vi "lab1.vi"() -> ()   [LabVIEW 2018]
uses:
  <vilib>/Utility/file.llb/Read Delimited Spreadsheet (DBL).vi
  <vilib>/Utility/file.llb/Write Delimited Spreadsheet (DBL).vi
panel:
  in  "Path 2":path
  in  "Path":path
  out "XY Graph":cluster{"all rows":dbl[], "all rows":dbl[]}[](graph)
  out "Waveform Graph 3":cluster{i32, i32, "all rows":dbl[]}(graph)
  out "Waveform Graph":cluster{i32, i32, "all rows":dbl[]}(graph)
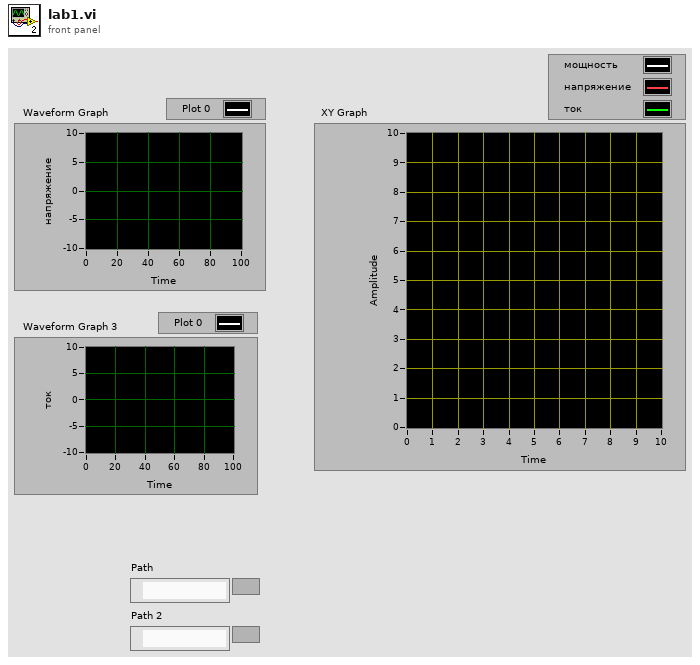
[diagram p1: front panel]
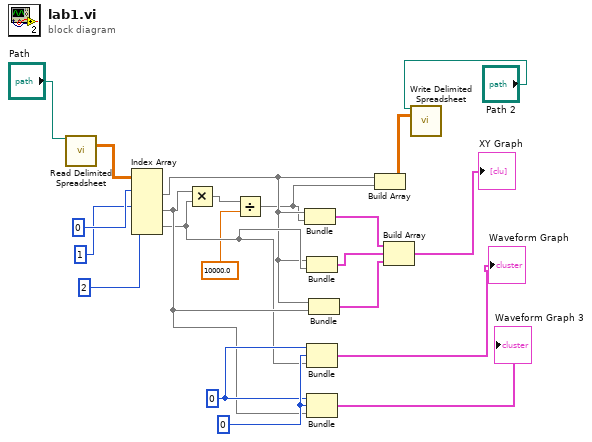
[diagram p0: block diagram]
diagram:
  w16 = 0
  w15 = 0
  n1 = call-poly <vilib>:"Read Delimited Spreadsheet.vi"("file path (dialog if empty)"="Path", "mark after read (chars.)"=w9) -> ("all rows"=w17:dbl[][], "EOF?"=w9:bool)  [unwired: 9 in, 3 out]
  n2 = Index Array(array=w17, index (row) #1=0, index (row) #2=1, index (row) #3=2) -> (element #1=w11:dbl[], element #2=w14:dbl[], element #3=w13:dbl[])  [unwired: 3 in]
  n3 = Multiply(x=w14, y=w13) -> (x*y=w22:dbl[])
  n4 = Divide(x=w22, y=10000.0) -> (x/y=w10:dbl[])
  n5 = Bundle("all rows"=w11, w10) -> (w6:cluster{"all rows":dbl[], dbl[]})  [unwired: 1 in]
  n6 = Bundle("all rows"=w11, "all rows"=w13) -> (w5:cluster{"all rows":dbl[], "all rows":dbl[]})  [unwired: 1 in]
  n7 = Bundle(w15, w16, "all rows"=w13) -> (→"Waveform Graph":cluster{i32, i32, "all rows":dbl[]})  [unwired: 1 in]
  n8 = Bundle(w15, w16, "all rows"=w14) -> (→"Waveform Graph 3":cluster{i32, i32, "all rows":dbl[]})  [unwired: 1 in]
  n9 = Bundle("all rows"=w11, "all rows"=w14) -> (w4:cluster{"all rows":dbl[], "all rows":dbl[]})  [unwired: 1 in]
  n10 = Build Array(w11, w10) -> (w8:dbl[][])
  n11 = Build Array(w6, w5, w4) -> (→"XY Graph":cluster{"all rows":dbl[], "all rows":dbl[]}[])
  n12 = call-poly <vilib>:"Write Delimited Spreadsheet.vi"("file path (dialog if empty)"="Path 2", "2D data"=w8) -> ()  [unwired: 12 in, 2 out]
